vi "PostError.vi"(8 "error in (no error)":errorcluster, 9 "Type":T1, 10 "Message":string, 11 "IErrorManager in":refnum<class "IErrorManager.lvclass">) -> (0 "error out":errorcluster, 3 "IErrorManager out":refnum<class "IErrorManager.lvclass">)   [LabVIEW 2020, in "LabVIEWObjectInterfaces.lvlib" / "IErrorManager.lvclass"]
uses:
  IErrorManager.lvclass
  ErrorManager/ErrorManager/ErrorType.ctl
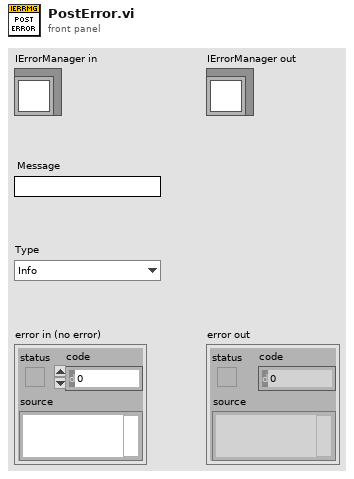
[diagram p1: front panel]
types:
  T1 = typedef "LabVIEWObjectInterfaces.lvlib/IErrorManager.lvclass/ErrorType.ctl" = enum16{"Info", "Warning", "Error"}
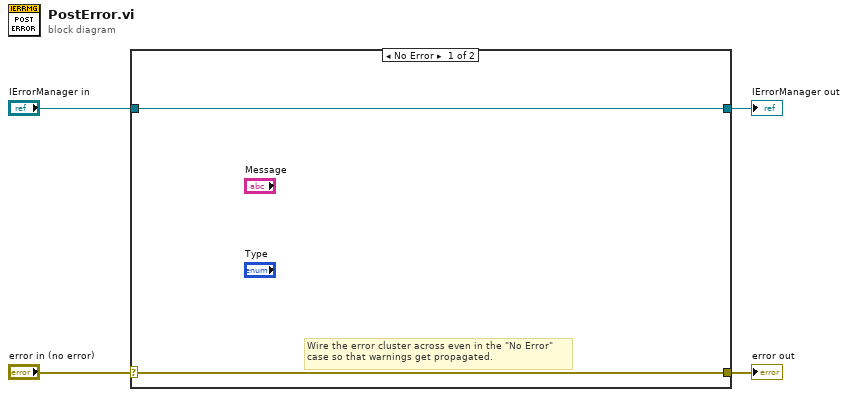
[diagram p0: block diagram]
diagram:
  n1 = case shown="No Error" "error in (no error)" {
    selector: "error in (no error)" -> [w5 w8]
    tunnel: [w5 w8] -> w3
    tunnel: [w6 w7] -> w1
    tunnel: "IErrorManager in" -> [w6 w7]
    frame No Error {
      # "Wire the error cluster across even in the \"No Error\"\ncase so that warnings get propagated."
    }
    frame Error {
    }
  }
  "error out" <- w3
  "IErrorManager out" <- w1
